vi "Launch Connection Handler.vi"(4 "error in (no error)":errorcluster, 6 "Debugging?":bool, 7 "TCP Network Connection in":refnum<k5>) -> (0 "error out":errorcluster)   [LabVIEW 2015, in "Startup Processes.lvlib"]
uses:
  Startup Processes.lvlib
  Custom TCP Connection Handler.vi
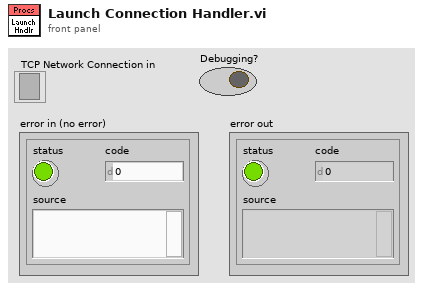
[diagram p1: front panel]
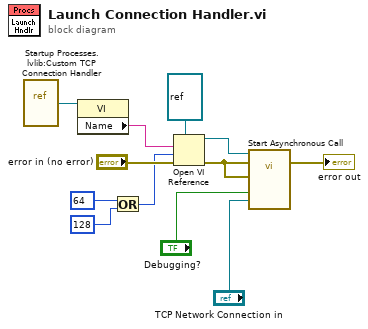
[diagram p0: block diagram]
diagram:
  n1 = vi-ref "Startup Processes.lvlib:Custom TCP Connection Handler.vi"() -> (w12:refnum<vi>)
  n2 = property class="VI"(reference=w12) -> ("Name"=w11:string)  [unwired: 1 in, 2 out]
  n3 = Or(x=64 ("options"), y=128 ("options")) -> (x .or. y?=w6:i32)
  n4 = Open VI Reference(type specifier VI Refnum (for type only)=refnum<vi> refnum, vi path=w11, options=w6, error in (no error)="error in (no error)") -> (vi reference=w5:refnum<vi>, error out=w3:errorcluster)  [unwired: 2 in]
  n5 = call-by-ref "Start Asynchronous Call"(reference=w5, error in=w3, "TCP Network Connection in"="TCP Network Connection in", "Debugging"="Debugging?", "Error In"=w3) -> (error out=→"error out":errorcluster)  [unwired: 4 in, 2 out]
